vi "LoadSyncMasterHW.vi"(8 "error in (no error)":errorcluster, 11 "BME_DG_System in":refnum<class "BME_DG_System.lvclass">) -> (0 "error out":errorcluster, 3 "BME_DG_System out":refnum<class "BME_DG_System.lvclass">)   [LabVIEW 2009, in "POLARIS BME DG.lvlib" / "BME_DG_System.lvclass"]
uses:
  BME_DG_System.lvclass
  BME_DG_Base/BME_DG_Base.lvclass
  POLARIS BME DG.lvlib
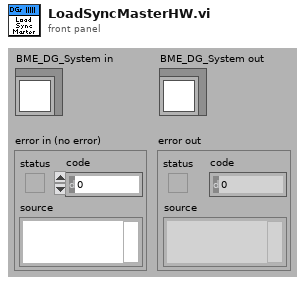
[diagram p1: front panel]
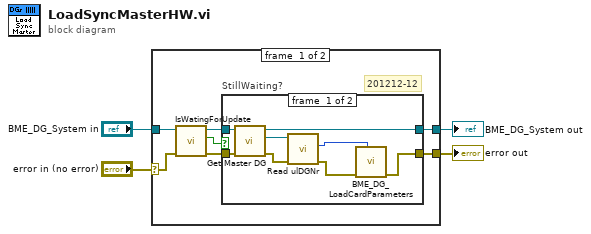
[diagram p0: block diagram]
diagram:
  n1 = case shown="No Error" "error in (no error)" {
    selector: "error in (no error)" -> [w8 w23]
    tunnel: [w10 w23] -> w3
    tunnel: [w11 w22] -> w1
    tunnel: "BME_DG_System in" -> [w9 w22]
    frame #0 {
      # "201212-12"
      n2 = call "IsWatingForUpdate.vi"("error in (no error)"=w8, "BME_DG_System in"=w9) -> ("error out"=w7:errorcluster, "StillWaiting"=w5:bool, "BME_DG_System out"=w6:refnum<class "BME_DG_System.lvclass">)  [unwired: 7 in]
      n3 = case "StillWaiting?" shown="False" w5 {
        tunnel: [w19 w21] -> w11
        tunnel: [w14 w20] -> w10
        tunnel: w7 -> [w13 w20]
        tunnel: w6 -> [w12 w21]
        frame #0 {
          n4 = call "Get Master DG.vi"("error in (no error)"=w13, "BME_DG_System in"=w12) -> ("error out"=w17:errorcluster, "BME_DG_Base.lvclass"=w18:refnum<class "BME_DG_Base.lvclass">, "BME_DG_System out"=w19:refnum<class "BME_DG_System.lvclass">)  [unwired: 6 in, 1 out]
          n5 = call-dynamic "Read ulDGNr.vi"("error in (no error)"=w17, "BME_DG_Base in"=w18) -> ("error out"=w16:errorcluster, "ulDGNr"=w15:u32)  [unwired: 6 in, 2 out]
          n6 = call "BME_DG_LoadCardParameters.vi"("DG_Number"=w15, "error in (no error)"=w16) -> ("error out"=w14:errorcluster)  [unwired: 9 in]
        }
        frame #1 {
        }
      }
    }
    frame #1 {
    }
  }
  "error out" <- w3
  "BME_DG_System out" <- w1
